vi "Encoder to Angle conversion.vi"(10 "Input":i64) -> (2 "Output":dbl)   [LabVIEW 2013, in "ProcessorHelperFunctions.lvlib"]
uses:
  ProcessorHelperFunctions.lvlib
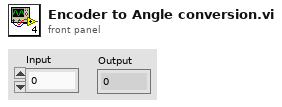
[diagram p1: front panel]
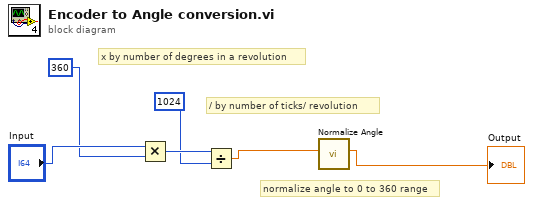
[diagram p0: block diagram]
diagram:
  # "normalize angle to 0 to 360 range"
  # "/ by number of ticks/ revolution"
  # "x by number of degrees in a revolution"
  n1 = Multiply(x="Input", y=360) -> (x*y=w6:i64)
  n2 = Divide(x=w6, y=1024) -> (x/y=w2:dbl)
  n3 = call "Normalize Angle.vi"("Input"=w2) -> ("Output"=→"Output":dbl)  [unwired: 10 in]
